vi "main_old.vi"() -> ()   [LabVIEW 2023]
uses:
  subVis/datas.ctl
  subVis/HologramInfo.ctl
  HoloPyLib/holoTracker.lvlib
  subVis/analyse_parameters.ctl
  <vilib>/Math Plots/3D Math Plots/3D Scatter/3D Scatter Datatype/3D Scatter Datatype.lvclass
  HoloPyLib/CCL_parameters.ctl
  HoloPyLib/parameters.ctl
  <vilib>/Math Plots/3D Math Plots/3D Scatter/3D Scatter Datatype/Public/Plot Helper (Vector).vi
  subVis/referencesBtns.ctl
  <vilib>/Math Plots/3D Math Plots/3D Scatter/3D Scatter XCtrl/3D Scatter.xctl
panel:
  out "Status":string
  in  "result tab":T1(tab)
  out "2D Picture":picture caption="Hologram"
  out "3D Scatter":refnum<class "3D Plot Datatype.lvclass">[](xcontrol)
  out "FEATURES":sgl[][](array[numeric])=[[0.0, 6.612585e-05, 1.9695788e-05, 1.0777613e-06, 1136.0], [0.0, 6.468655e-05, 2.2335455e-05, 1.0884105e-05, 10108.0], [0.0, 0.00015315457, 2.5819925e-05, 6.314848e-06, 8098.0], [0.0, 0.00014578222, 2.5758109e-05, 6.202794e-06, 6254.0], [0.0, 5.3788557e-05, 4.846046e-05, 1.6199401e-06, 4030.0], [0.0, 4.554296e-05, 5.2554697e-05, 2.3448233e-06, 5183.0], [0.0, 6.719615e-05, 0.00010475709, 9.479025e-06, 45705.0], [0.0, 0.0001519142, 0.000113882794, 3.5307496e-06, 7166.0], [0.0, 0.00014522657, 0.000117954936, 1.656648e-06, 2687.0], [0.0, 0.0001657626, 0.00017647912, 6.7820397e-06, 22008.0], [0.0, 0.0001543048, 0.00017526228, 4.2125926e-06, 4890.0], [0.0, 0.000108675, 0.00016782495, 4.2502693e-06, 6.0], [0.0, 5.2179905e-05, 4.8786325e-05, 1.0611426e-05, 896.0], [0.0, 7.633682e-05, 0.00010101719, 1.2997062e-05, 980.0], [0.0, 0.0001484, 0.000117425, 1.25e-05, 1.0], [0.0, 0.0001485656, 0.000115037496, 1.34489665e-05, 57.0], [0.0, 0.00014867843, 0.00011536141, 2.0105621e-05, 9059.0], [0.0, 4.993365e-05, 5.1556737e-05, 3.0146293e-05, 17286.0], [0.0, 0.00014947906, 2.572066e-05, 2.6544916e-05, 9378.0], [0.0, 3.406486e-05, 1.555056e-05, 3.0145982e-05, 9879.0], [0.0, 0.00014836973, 0.00013649464, 2.4943547e-05, 115.0], [0.0, 0.00010474305, 0.000167082, 3.4538934e-05, 11030.0], [0.0, 0.00016031138, 0.00017643355, 4.1315438e-05, 26224.0], [0.0, 4.673895e-05, 0.00013298314, 3.0840518e-05, 1181.0], [0.0, 4.4124776e-05, 0.000131255, 3.0545714e-05, 187.0], [0.0, 6.8812704e-05, 7.23215e-05, 3.4768887e-05, 4117.0], [0.0, 9.791127e-05, 5.2118266e-06, 3.6847057e-05, 2200.0], [0.0, 0.00017519953, 0.00015975515, 3.4322784e-05, 1209.0], [0.0, 0.00013256604, 3.5334786e-05, 3.941026e-05, 808.0], [0.0, 0.00013814989, 9.710776e-05, 3.901609e-05, 65.0], [0.0, 0.00016371529, 4.329701e-05, 4.3546614e-05, 2335.0]]
  in  "Tab Control":T2(tab)=enum."ACTIONS"
  in  "Holograms directory":path=path "C:/TRAVAIL/developpement/imagesHolo/1000im_manip3"
  in  "Test hologram path":path=path "C:/TRAVAIL/developpement/imagesHolo/1000im_manip3/100um_40x_int_.7ajmvz4e.000000.bmp"
  in  "Python version":string="3.10"
  in  "Analyse parameters":T3={"propagation"={"distance ini"=0.0, "number of planes"=200, "step"=5e-07, "Fourier BP filter (pix)"={"High pass (0=none)"=15.0, "Low Pass (0=none)"=125.0}}, "Focus"={"Type"=enum."SUM_OF_VARIANCE", "Sum size"=15}, "Remove mean Hologram"=FALSE, "CCL parameters"={"Threshold ( N x Standard deviation)"=10.0, "Connectivity"=enum."26", "min voxel"=1.0, "max voxel"=0.0}} {"CCL parameters"."max voxel" min=0.0 max=0.0; "CCL parameters"."min voxel" min=1.0 max=100.0; "CCL parameters"."Threshold ( N x Standard deviation)" min=1.0 max=100.0; "Focus"."Sum size" min=1 max=100; "propagation"."Fourier BP filter (pix)"."Low Pass (0=none)" format="%#_6f"; "propagation"."step" format="%#_6e"; "propagation"."distance ini" format="%#_6e"}
  in  "Holo parameters":T5={"wavelength"=6.6e-07, "optical index"=1.33, "Holo size X"=1024, "Holo size Y"=1024, "pixel size"=7e-06, "objective magnification"=40.0} {"wavelength" format="%#_6e"}
  in  "CANCEL_BATCH":bool
  in  "Batch parameters":T6
  in  "EXIT":bool
  in  "close HOLO":bool
  in  "findFeatures":bool
  in  "reconstruct&Focus":bool
  in  "removeMeanHolo":bool
  in  "openHOLO":bool
  in  "BATCH":bool
  out "dt(ms)":u32=190105
  in  "display\nsub-volume\n3 planes":bool
  in  "display_XY_SUM":bool
  in  "display_XZ_SUM":bool
  in  "display_YZ_SUM":bool
  in  "displayBinPlane":bool
  in  "TEST SUM BIN PLANE":bool
  in  "Plane number":u16=95
  in  "displayPlane":bool
  in  "displayXYMax":bool
  in  "displayXZMax":bool
  in  "displayYZMax":bool
  in  "displayHolo":bool
  in  "param":T7
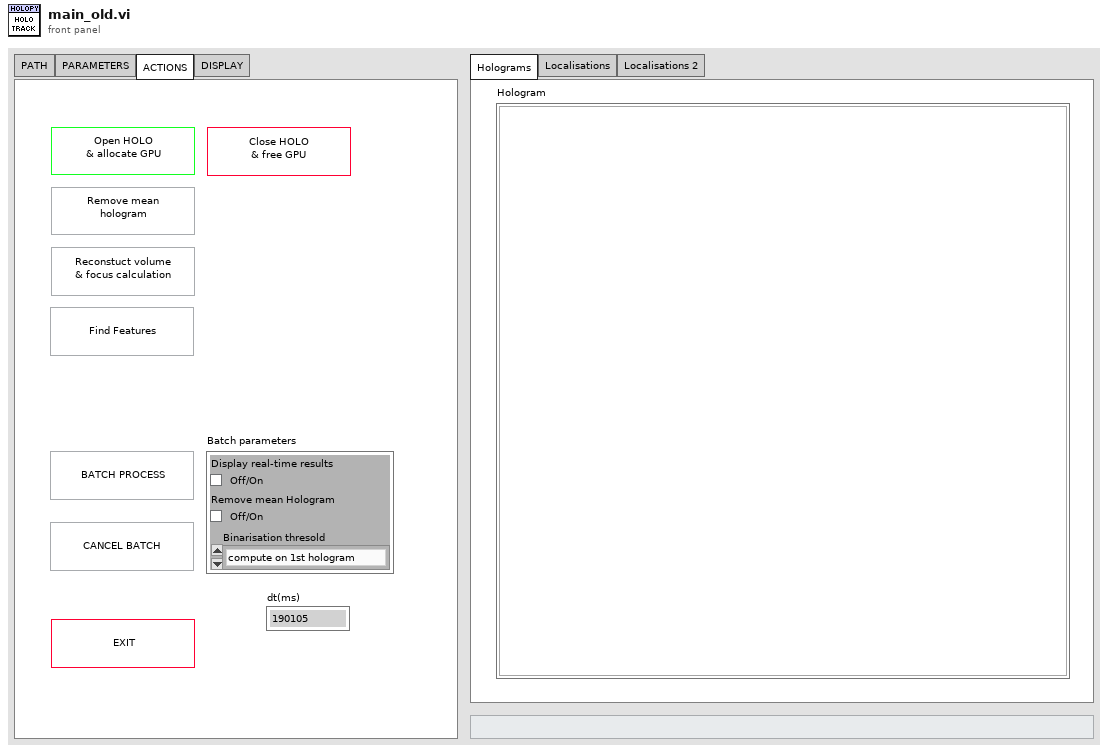
[diagram p1: front panel]
types:
  T1 = enum32{"Holograms", "Localisations", "Localisations 2"}
  T2 = enum32{"PATH", "PARAMETERS", "ACTIONS", "DISPLAY"}
  T3 = typedef "holoTracker.lvlib/analyse_parameters.ctl" = cluster{"propagation":cluster{"distance ini":dbl, "number of planes":i32, "step":dbl, "Fourier BP filter (pix)":cluster{"High pass (0=none)":dbl, "Low Pass (0=none)":dbl}}, "Focus":cluster{"Type":enum16{"SUM_OF_INTENSITY", "SUM_OF_LAPLACIAN", "SUM_OF_VARIANCE", "TENENGRAD"}, "Sum size":i32}, "Remove mean Hologram":bool, "CCL parameters":T4}
  T4 = typedef "CCL_parameters.ctl" = cluster{"Threshold ( N x Standard deviation)":dbl, "Connectivity":enum16{"6", "18", "26"}, "min voxel":dbl, "max voxel":dbl}
  T5 = typedef "holoTracker.lvlib/HologramInfo.ctl" = cluster{"wavelength":sgl, "optical index":sgl, "Holo size X":i32, "Holo size Y":i32, "pixel size":sgl, "objective magnification":sgl}
  T6 = cluster{"Display real-time results":bool, "Remove mean Hologram":bool, "Binarisation thresold ":enum16{"compute on 1st hologram", "compute on each hologram"}}
  T7 = cluster{"X":i32, "Y":i32, "Z":i32, "XYsize":i32, "ZSize":i32}
  T8 = typedef "referencesBtns.ctl" = cluster{"PythonVer":refnum<vi>, "Python/Environnement\npath":refnum<vi>, "HoloPath":refnum<vi>, "HoloDir":refnum<vi>, "Holo parameters":refnum<vi>, "Remove mean Hologram":refnum<vi>, "propagation":refnum<vi>, "Fourier BP filter (pix)":refnum<vi>, "Focus":refnum<vi>, "Batch thresold ":refnum<vi>, "CCL parameters":refnum<vi>, "testMode":refnum<vi>, "exitTestMode":refnum<vi>, "BATCH":refnum<vi>, "CANCEL_BATCH":refnum<vi>, "EXIT":refnum<vi>, "Plane number":refnum<vi>, "Display":refnum<vi>}
  T9 = typedef "datas.ctl" = cluster{"PythonSession":refnum<k35>, "Display":bool, "BinThreshold":sgl, "LIST HOLO BATCH":path[], "Display":sgl[][], "meanHolo":sgl[][], "FEATURES(µm)":sgl[][], "LabelPicture":string, "Status":string, "planeToDisplayFeatures":enum16{"XY", "XZ", "YZ"}, "State":enum16{"SESSION CLOSED", "WAIT", "TEST WAIT", "TEST IN PROGESS", "BATCH IN PROGRESS"}}
  T10 = typedef "parameters.ctl" = cluster{"Holo parameters":T5, "Analyse parameters":T3}
  T11 = cluster{"Test hologram path":path, "Display?":bool}
  T12 = cluster{"allocated?":bool, "reconstructed?":bool, "BATCH?":bool}
  T13 = cluster{"Holo":sgl[][], "XYFeatures(pix)":sgl[][], "FEATURES(µm)":sgl[][]}
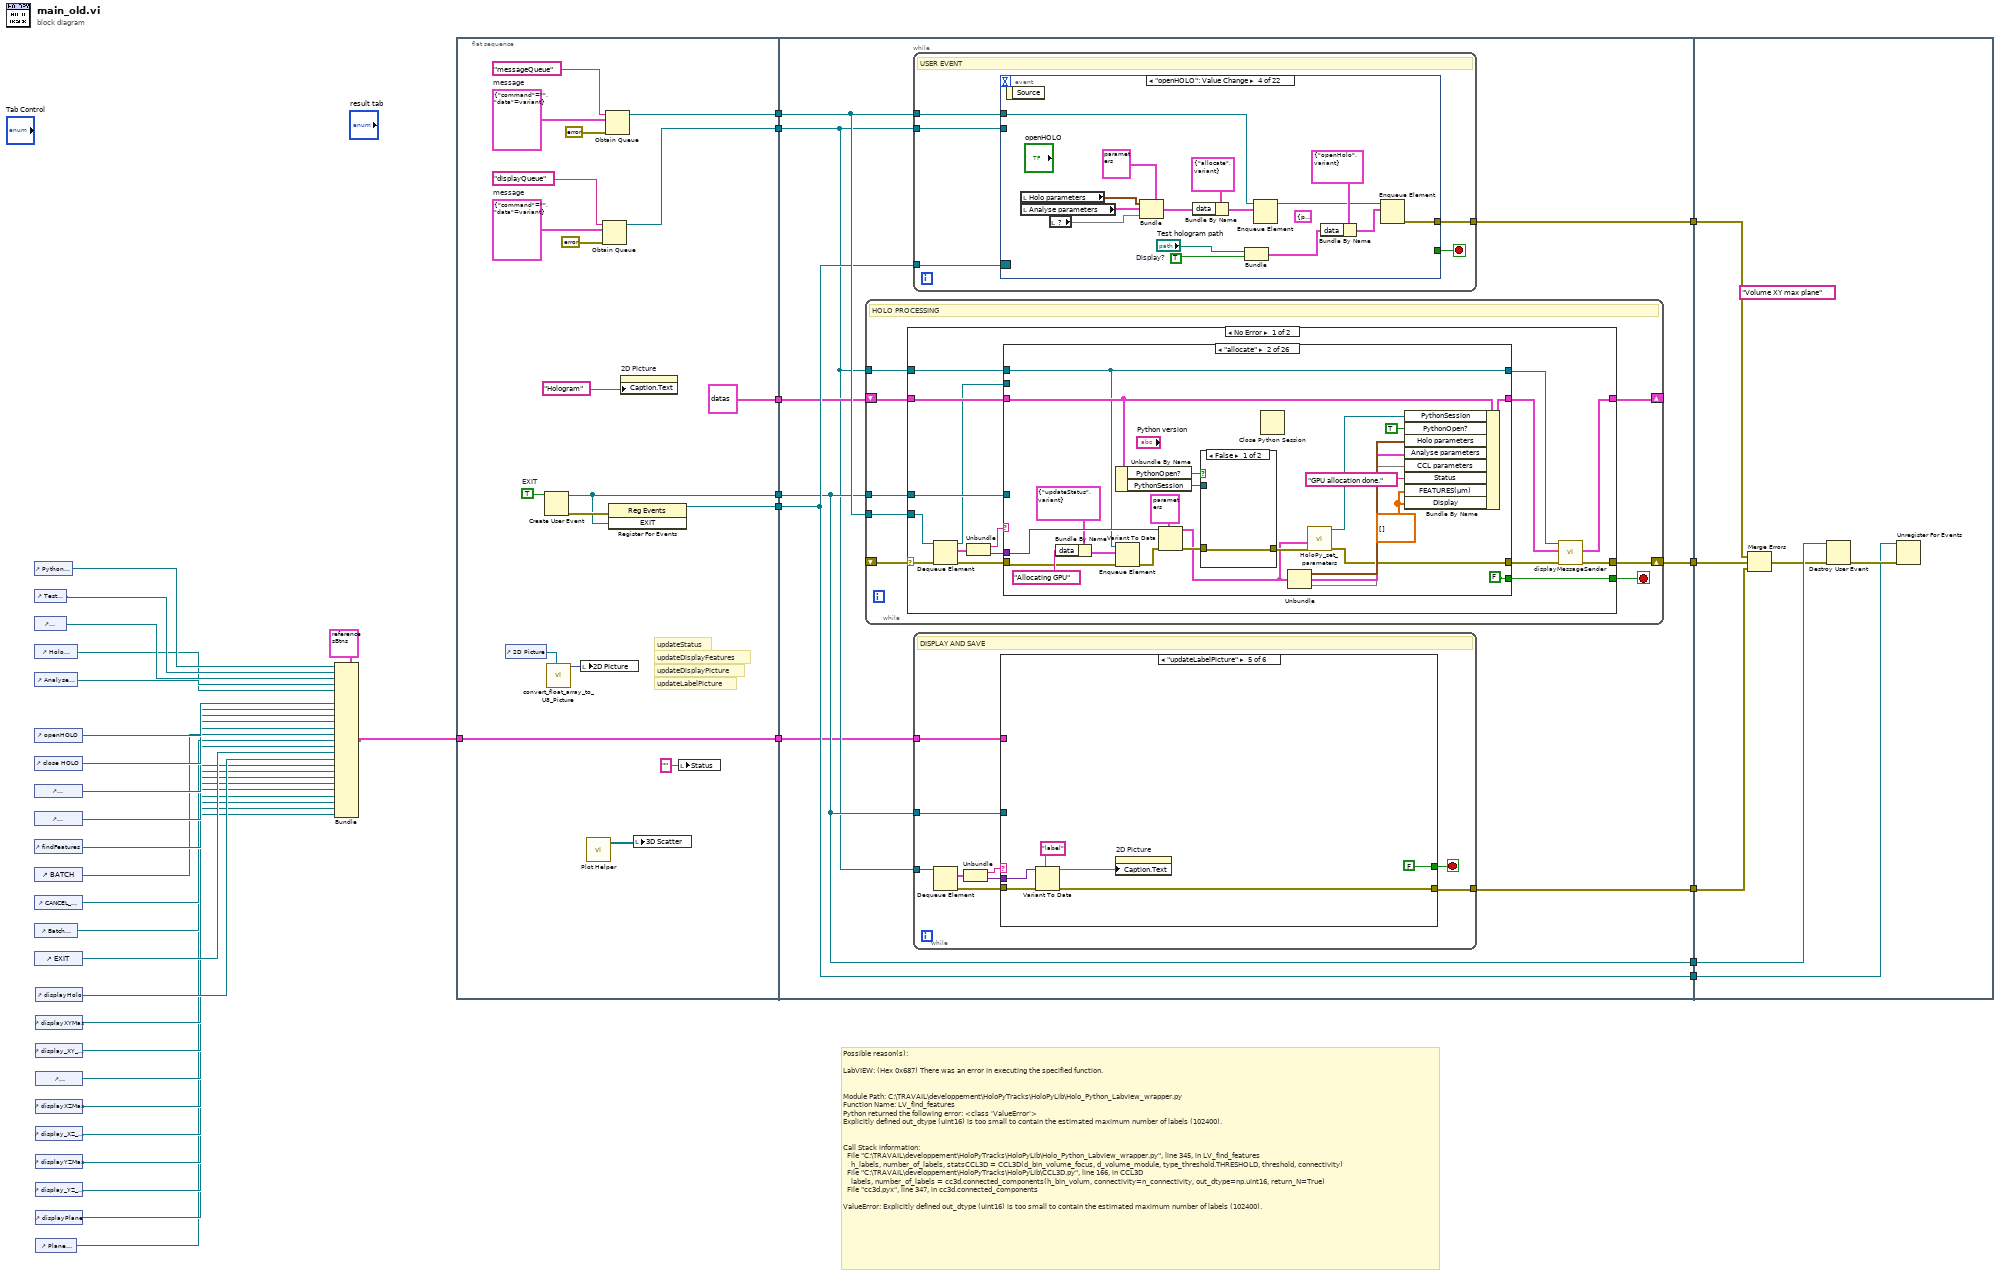
[diagram p0: block diagram]
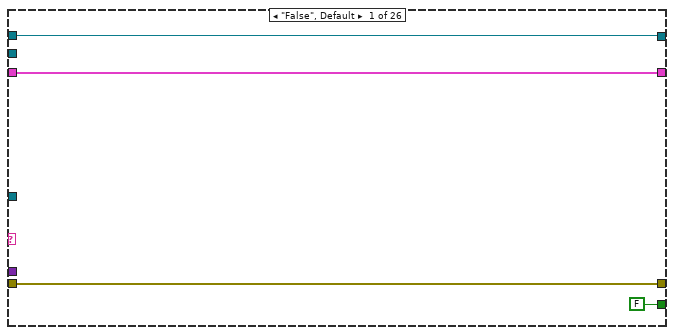
[diagram p2: hidden frame]
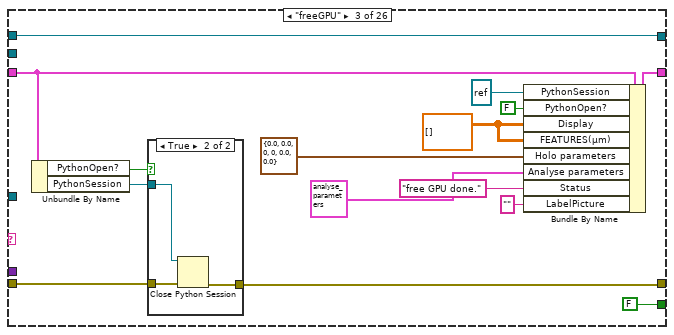
[diagram p4: hidden frame]
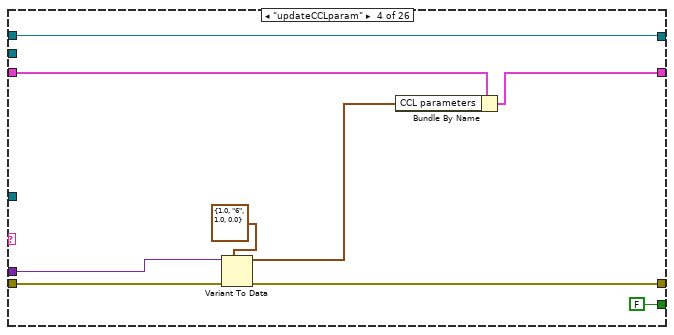
[diagram p6: hidden frame]
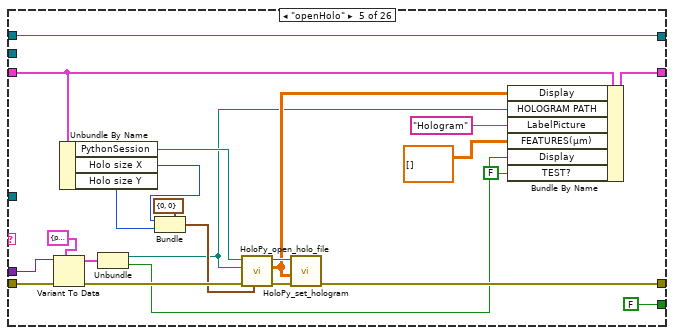
[diagram p7: hidden frame]
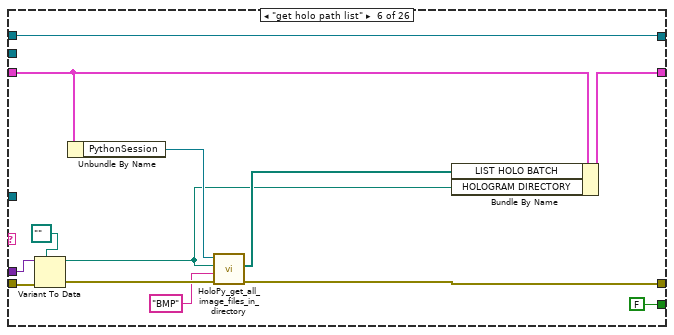
[diagram p8: hidden frame]
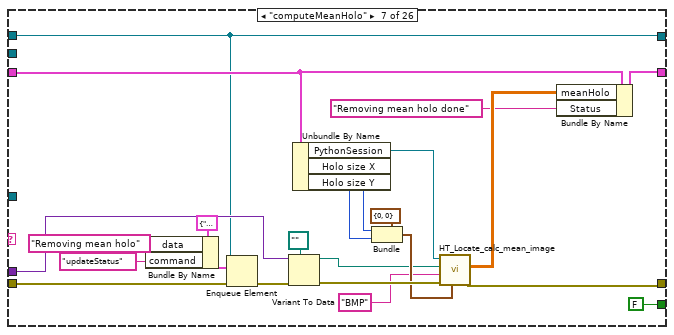
[diagram p9: hidden frame]
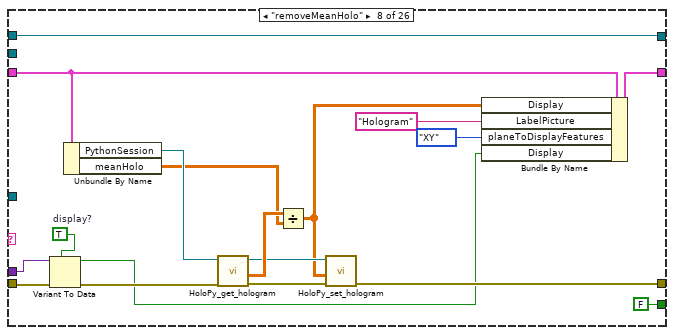
[diagram p10: hidden frame]
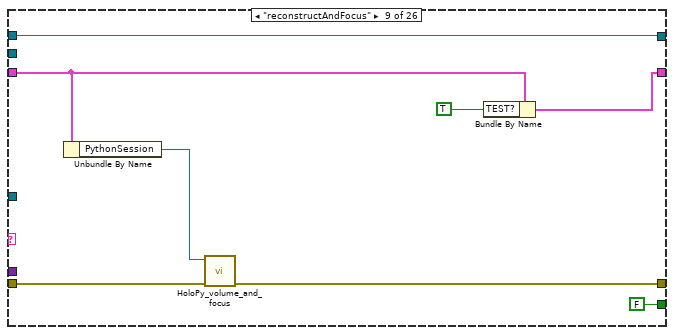
[diagram p11: hidden frame]
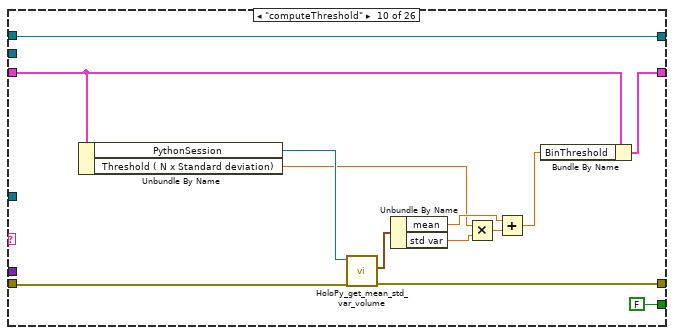
[diagram p12: hidden frame]
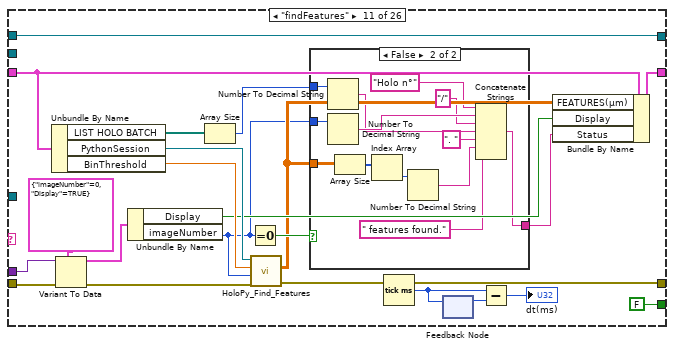
[diagram p13: hidden frame]
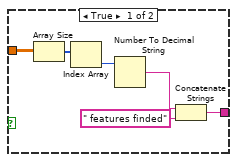
[diagram p14: hidden frame]
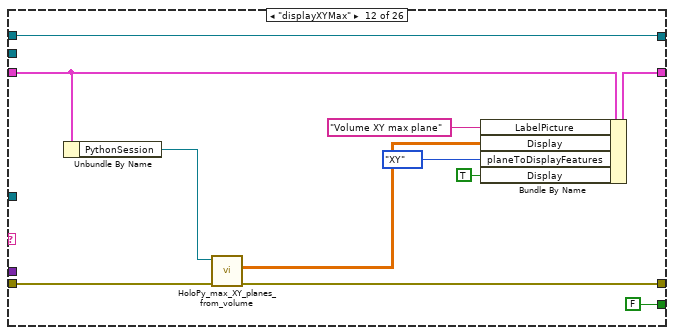
[diagram p15: hidden frame]
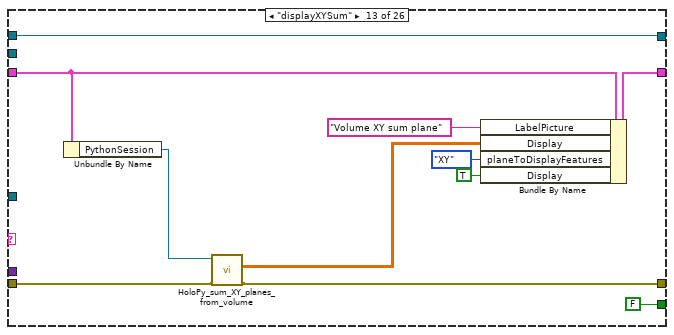
[diagram p16: hidden frame]
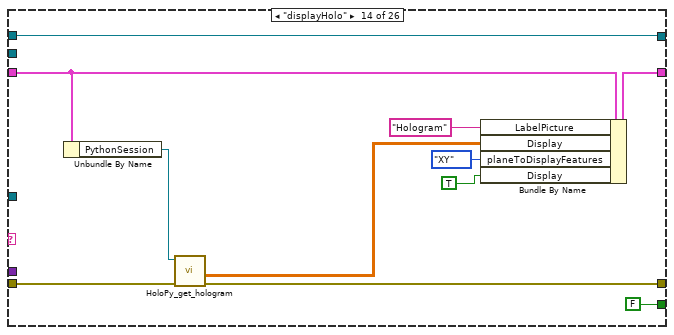
[diagram p17: hidden frame]
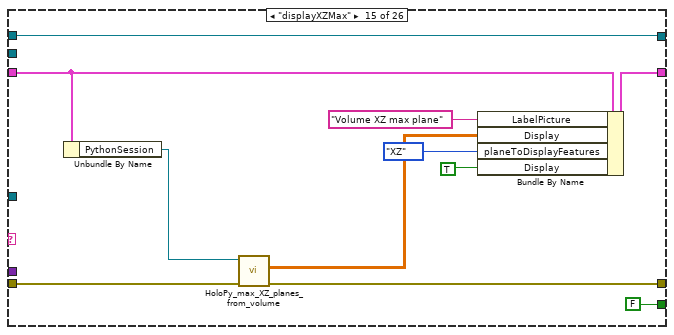
[diagram p18: hidden frame]
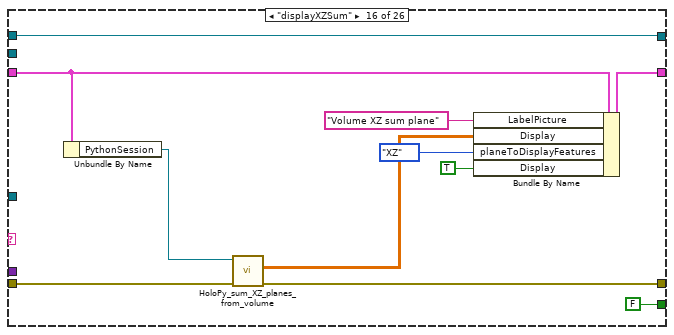
[diagram p19: hidden frame]
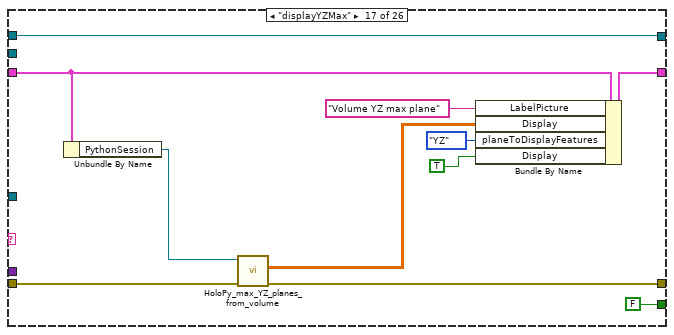
[diagram p20: hidden frame]
diagram:
  # "Possible reason(s):\n\nLabVIEW: (Hex 0x687) There was an error in executing the specified function.\n\n\nModule Path: C:\\TRAVAIL\\developpement\\HoloPyTracks\\HoloPyLib\\Holo_Python_Labview_wrapper.py\nFunction Name: LV_find_features\nPython returned the following error: <class 'ValueError'>\nExplicitly defined out_dtype (uint16) is too small to contain the estimated maximum number of labels (102400).\n\n\nCall Stack information:\n  File \"C:\\TRAVAIL\\developpement\\HoloPyTracks\\HoloPyLib\\Holo_Python_Labview_wrapper.py\", line 345, in LV_find_features\n    h_labels, number_of_labels, statsCCL3D = CCL3D(d_bin_volume_focus, d_volume_module, type_threshold.THRESHOLD, threshold, connectivity)\n  File \"C:\\TRAVAIL\\developpement\\HoloPyTracks\\HoloPyLib\\CCL3D.py\", line 166, in CCL3D\n    labels, number_of_labels = cc3d.connected_components(h_bin_volum, connectivity=n_connectivity, out_dtype=np.uint16, return_N=True)\n  File \"cc3d.pyx\", line 347, in cc3d.connected_components\n\nValueError: Explicitly defined out_dtype (uint16) is too small to contain the estimated maximum number of labels (102400)."
  n1 = control-ref of="Python version"() -> (w28:refnum<vi>)
  n2 = control-ref of="Test hologram path"() -> (w27:refnum<vi>)
  n3 = control-ref of="Holograms directory"() -> (w26:refnum<vi>)
  n4 = control-ref of="Holo parameters"() -> (w25:refnum<vi>)
  n5 = control-ref of="Analyse parameters"() -> (w24:refnum<vi>)
  n6 = control-ref of="openHOLO"() -> (w22:refnum<vi>)
  n7 = control-ref of="close HOLO"() -> (w21:refnum<vi>)
  n8 = control-ref of="removeMeanHolo"() -> (w20:refnum<vi>)
  n9 = control-ref of="reconstruct&Focus"() -> (w19:refnum<vi>)
  n10 = control-ref of="findFeatures"() -> (w18:refnum<vi>)
  n11 = control-ref of="BATCH"() -> (w17:refnum<vi>)
  n12 = control-ref of="CANCEL_BATCH"() -> (w16:refnum<vi>)
  n13 = control-ref of="Batch parameters"() -> (w15:refnum<vi>)
  n14 = control-ref of="EXIT"() -> (w14:refnum<vi>)
  n15 = control-ref of="displayHolo"() -> (w13:refnum<vi>)
  n16 = control-ref of="displayXYMax"() -> (w12:refnum<vi>)
  n17 = control-ref of="display_XY_SUM"() -> (w11:refnum<vi>)
  n18 = control-ref of="displayBinPlane"() -> (w10:refnum<vi>)
  n19 = control-ref of="displayXZMax"() -> (w9:refnum<vi>)
  n20 = control-ref of="display_XZ_SUM"() -> (w8:refnum<vi>)
  n21 = control-ref of="displayYZMax"() -> (w7:refnum<vi>)
  n22 = control-ref of="display_YZ_SUM"() -> (w6:refnum<vi>)
  n23 = control-ref of="displayPlane"() -> (w5:refnum<vi>)
  n24 = control-ref of="Plane number"() -> (w4:refnum<vi>)
  n25 = Bundle(cluster=T8 {"PythonVer"=refnum, "Python/Environnement\npath"=refnum, "HoloPath"=refnum, "HoloDir"=refnum, "Holo parameters"=refnum, "Remove mean Hologram"=refnum, "propagation"=refnum, "Fourier BP filter (pix)"=refnum, "Focus"=refnum, "Batch thresold "=refnum, "CCL parameters"=refnum, "testMode"=refnum, "exitTestMode"=refnum, "BATCH"=refnum, "CANCEL_BATCH"=refnum, "EXIT"=refnum, "Plane number"=refnum, "Display"=refnum} ("output cluster"), w28, w27, w26, w25, w24, w22, w21, w20, w19, w18, w17, w16, w15, w14, w13, w12, w11, w10, w9, w8, w7, w6, w5, w4) -> (w1:T8, w23:refnum<vi>)
  n26 = flat-sequence {
    tunnel: [w55] -> w38
    tunnel: [w51] -> w37
    tunnel: [w50] -> w36
    tunnel: [w46] -> w35
    tunnel: [T9 {"PythonSession"=refnum, "Display"=FALSE, "BinThreshold"=0.0, "LIST HOLO BATCH"=[], "Display"=[], "meanHolo"=[], "FEATURES(µm)"=[], "LabelPicture"="", "Status"="", "planeToDisplayFeatures"=enum."XY", "State"=enum."WAIT"}] -> w34
    tunnel: [w39] -> w2
    tunnel: w1 -> [w39]
    tunnel: w38 -> [w66]
    tunnel: w37 -> [w63]
    tunnel: w36 -> [w65]
    tunnel: w35 -> [w61]
    tunnel: w34 -> [w62]
    tunnel: [w65] -> w33
    tunnel: [w63] -> w32
    tunnel: [w64] -> w31
    tunnel: [w60] -> w30
    tunnel: [w59] -> w29
    tunnel: w2 -> [w58]
    tunnel: w33 -> [w695]
    tunnel: w32 -> [w694]
    tunnel: w31 -> [w691]
    tunnel: w30 -> [w693]
    tunnel: w29 -> [w692]
    frame #0 {
      w48 = cluster{"command":string, "data":variant} {"command"="", "data"=variant}  # message
      w53 = TRUE  # EXIT
      w56 = cluster{"command":string, "data":variant} {"command"="", "data"=variant}  # message
      # "updateDisplayFeatures"
      # "updateLabelPicture"
      # "updateDisplayPicture"
      # "updateStatus"
      n27 = control-ref of="2D Picture"() -> (w44:refnum<vi>)
      n28 = Create User Event(user event datatype=w53) -> (user event=w51:refnum<user-event>, error out=w52:errorcluster)  [unwired: 1 in]
      n29 = call "convert_float_array_to_U8_Picture.vi"("Pict Refnum"=w44) -> ("new picture"=w43:picture)  [unwired: 9 in, 1 out]
      n30 = local write "2D Picture"(w43) -> ()
      n31 = call-poly <vilib>:"Plot Helper.vi"() -> ("3D Plot lvclass Array out"=w40:refnum<class "3D Plot Datatype.lvclass">[])  [unwired: 6 in, 5 out]
      n32 = Obtain Queue(name (unnamed)="displayQueue", element data type=w48, error in (no error)=errorcluster {"status"=FALSE, "code"=0, "source"=""}) -> (queue out=w46:refnum<queue>)  [unwired: 2 in, 2 out]
      n33 = Obtain Queue(name (unnamed)="messageQueue", element data type=w56, error in (no error)=errorcluster {"status"=FALSE, "code"=0, "source"=""}) -> (queue out=w55:refnum<queue>)  [unwired: 2 in, 2 out]
      n34 = register-events(error in=w52, w51) -> (reference out=w50:refnum<event-registration>)  [unwired: 1 in, 1 out]
      n35 = property on="2D Picture" class="Pict"("Caption.Text"="Hologram" ("Label.Text")) -> ()  [unwired: 2 in, 2 out]
      n36 = local write "3D Scatter"(w40) -> ()
      n37 = local write "Status"("" ("Status")) -> ()
    }
    frame #1 {
      n38 = while {
        tunnel: w66 -> [w74]
        tunnel: w63 -> [w72]
        shift-right: [w70] -> _
        shift-left: w62 -> [w71]
        tunnel: w61 -> [w69]
        shift-right: [w68] -> w59
        shift-left: _ -> [w67]
        stop <- w73 stop-if-true
        # "HOLO PROCESSING"
        n39 = case shown="No Error" w67 {
          selector: w67 -> [w80 w489]
          tunnel: w74 -> [w90 w490]
          tunnel: [w85 FALSE] -> w73
          tunnel: w72 -> [w84 _]
          tunnel: w71 -> [w83 w485]
          tunnel: [w75 w485] -> w70
          tunnel: w69 -> [w82 _]
          tunnel: [w77 errorcluster {"status"=FALSE, "code"=0, "source"=""} ("error out")] -> w68
          frame No Error {
            n40 = Dequeue Element(queue=w90, error in (no error)=w80) -> (queue out=w81:refnum<queue>, element=w88:cluster{"command":string, "data":variant}, error out=w89:errorcluster)  [unwired: 1 in, 1 out]
            n41 = Unbundle(w88) -> ("command"=w87:string, "data"=w86:variant)
            n42 = case shown="\"allocate\"" w87 {
              tunnel: w89 -> [w92 w98 w128 w146 w169 w182 w190 w211 w231 w239 w266 w296 w302 w313 w324 w335 w346 w357 w369 w394 w411 w415 w433 w443 w467 w476]
              tunnel: w86 -> [_ w117 _ w145 w168 w181 w205 w210 _ _ w265 _ _ _ _ _ _ _ w368 w393 w410 _ w432 _ w466 _]
              tunnel: [FALSE FALSE FALSE FALSE FALSE FALSE FALSE FALSE FALSE FALSE FALSE FALSE FALSE FALSE FALSE FALSE FALSE FALSE FALSE FALSE FALSE FALSE FALSE FALSE FALSE TRUE] -> w85
              tunnel: w84 -> [_ _ _ _ _ _ _ _ _ _ _ _ _ _ _ _ _ _ _ _ _ _ _ _ _ w479]
              tunnel: w83 -> [w93 w115 w132 w142 w161 w179 w197 w218 w227 w237 w257 w292 w306 w317 w328 w339 w350 w361 w376 w389 w409 w422 w425 w451 w460 w471]
              tunnel: [w93 w116 w133 w141 w160 w180 w196 w216 w226 w236 w255 w291 w305 w316 w327 w338 w349 w360 w375 w388 w408 w421 w424 w452 w460 w470] -> w79
              tunnel: w82 -> [w91 w96 w122 w139 w153 w171 w184 w215 w229 w233 w258 w294 w307 w318 w329 w340 w351 w362 w377 w387 w407 w420 w427 w441 w458 w472]
              tunnel: [w92 w103 w124 w143 w151 w174 w186 w214 w228 w238 w256 w293 w299 w312 w321 w334 w345 w356 w372 w381 w398 w419 w429 w438 w463 w473] -> w76
              tunnel: w81 -> [_ _ _ _ _ _ _ _ _ _ _ _ _ _ _ _ _ _ _ _ _ _ w434 w444 _ _]
              tunnel: [w91 w96 w122 w139 w153 w171 w184 w215 w229 w233 w258 w294 w307 w318 w329 w340 w351 w362 w377 w387 w407 w420 w427 w441 w458 w472] -> w78
              frame "False", Default {
              }
              frame "allocate" {
                w101 = sgl[][] [] ("FEATURES(µm)")
                n43 = Bundle By Name(cluster=cluster{"command":string, "data":variant} {"command"="updateStatus", "data"=variant} ("element"), "data"="Allocating GPU" ("command")) -> (w95:cluster{"command":string, "data":variant})
                n44 = Unbundle By Name(w115) -> ("PythonOpen?"=w113:bool, "PythonSession"=w112:refnum<k35>)
                n45 = Enqueue Element(queue=w96, element=w95, error in (no error)=w98) -> (error out=w97:errorcluster)  [unwired: 1 in, 2 out]
                n46 = Variant To Data(error in=w97, type=T10 {"Holo parameters"={"wavelength"=0.0, "optical index"=0.0, "Holo size X"=0, "Holo size Y"=0, "pixel size"=0.0, "objective magnification"=0.0}, "Analyse parameters"={"propagation"={"distance ini"=0.0, "number of planes"=0, "step"=0.0, "Fourier BP filter (pix)"={"High pass (0=none)"=0.0, "Low Pass (0=none)"=0.0}}, "Focus"={"Type"=enum."SUM_OF_INTENSITY", "Sum size"=0}, "Remove mean Hologram"=FALSE, "CCL parameters"={"Threshold ( N x Standard deviation)"=10.0, "Connectivity"=enum."26", "min voxel"=1.0, "max voxel"=0.0}}} ("Parameters"), Variant=w117) -> (data=w105:T10, error out=w114:errorcluster)
                n47 = case shown="False" w113 {
                  tunnel: w114 -> [w119 _]
                  tunnel: w112 -> [_ _]
                  tunnel: [w119 _] -> w111
                  frame False {
                  }
                  frame True {
                  }
                }
                n48 = Close Python Session() -> ()  [unwired: 2 in, 1 out]
                n49 = Unbundle(w105) -> (w108:T5, w107:T3, w104)
                n50 = call "HoloPy_set_parameters.vi"("error in (no error)"=w111, 9:w105) -> ("error out"=w103:errorcluster, "Refnum out"=w110:refnum<k35>)  [unwired: 7 in, 1 out]
                n51 = Bundle By Name(cluster=w115, "PythonSession"=w110, "PythonOpen?"=TRUE ("allocated?"), "Holo parameters"=w108, "Analyse parameters"=w107, "CCL parameters"=w104, "Status"="GPU allocation done." ("command"), "FEATURES(µm)"=w101, "Display"=w101) -> (w116:T9)
              }
              frame "freeGPU" {
                w120 = sgl[][] [] ("Holo")
                n52 = Unbundle By Name(w132) -> ("PythonOpen?"=w131:bool, "PythonSession"=w130:refnum<k35>)
                n53 = case shown="True" w131 {
                  tunnel: w128 -> [w135 w138]
                  tunnel: w130 -> [_ w137]
                  tunnel: [w135 w136] -> w124
                  frame False {
                  }
                  frame True {
                    n54 = Close Python Session(session in=w137, error in=w138) -> (11:w136:errorcluster)
                  }
                }
                n55 = Bundle By Name(cluster=w132, "PythonSession"=refnum<k35> refnum, "PythonOpen?"=FALSE ("allocated?"), "Display"=w120, "FEATURES(µm)"=w120, "Holo parameters"=T5 {"wavelength"=0.0, "optical index"=0.0, "Holo size X"=0, "Holo size Y"=0, "pixel size"=0.0, "objective magnification"=0.0}, "Analyse parameters"=T3 {"propagation"={"distance ini"=0.0, "number of planes"=0, "step"=0.0, "Fourier BP filter (pix)"={"High pass (0=none)"=0.0, "Low Pass (0=none)"=0.0}}, "Focus"={"Type"=enum."SUM_OF_INTENSITY", "Sum size"=1}, "Remove mean Hologram"=FALSE, "CCL parameters"={"Threshold ( N x Standard deviation)"=10.0, "Connectivity"=enum."26", "min voxel"=1.0, "max voxel"=0.0}}, "Status"="free GPU done." ("command"), "LabelPicture"="" ("command")) -> (w133:T9)
              }
              frame "updateCCLparam" {
                n56 = Variant To Data(error in=w146, type=T4 {"Threshold ( N x Standard deviation)"=1.0, "Connectivity"=enum."6", "min voxel"=1.0, "max voxel"=0.0} ("CCL parameters"), Variant=w145) -> (data=w140:T4, error out=w143:errorcluster)
                n57 = Bundle By Name(cluster=w142, "CCL parameters"=w140) -> (w141:T9)
              }
              frame "openHolo" {
                n58 = Variant To Data(error in=w169, type=T11 {"Test hologram path"=path "", "Display?"=FALSE} ("openHolo"), Variant=w168) -> (data=w155:T11, error out=w166:errorcluster)
                n59 = Unbundle By Name(w161) -> ("PythonSession"=w167:refnum<k35>, "Holo size X"=w163:i32, "Holo size Y"=w162:i32)
                n60 = Unbundle(w155) -> ("Test hologram path"=w154:path, "Display?"=w149:bool)
                n61 = Bundle(cluster=cluster{"image_size_X":i32, "image_size_Y":i32} {"image_size_X"=0, "image_size_Y"=0} ("imageSize"), "image_size_X"=w163, "image_size_Y"=w162) -> (w164:cluster{"image_size_X":i32, "image_size_Y":i32})
                n62 = call "HoloPy_open_holo_file.vi"("imageSize"=w164, "error in (no error)"=w166, "image path"=w154, "Refnum in"=w167) -> ("error out"=w159:errorcluster, "Array"=w157:sgl[][], "Refnum out"=w158:refnum<k35>)  [unwired: 5 in]
                n63 = call "HoloPy_set_hologram.vi"("error in (no error)"=w159, "HOLO_array"=w157, "Refnum in"=w158) -> ("error out"=w151:errorcluster)  [unwired: 6 in, 2 out]
                n64 = Bundle By Name(cluster=w161, "Display"=w157, "HOLOGRAM PATH"=w154, "LabelPicture"="Hologram" ("Label.Text"), "FEATURES(µm)"=sgl[][] [], "Display"=w149, "TEST?"=FALSE ("reconstructed?")) -> (w160:T9)
              }
              frame "get holo path list" {
                n65 = Variant To Data(error in=w182, type=path "" ("Holograms directory"), Variant=w181) -> (data=w173:path, error out=w178:errorcluster)
                n66 = Unbundle By Name(w179) -> ("PythonSession"=w177:refnum<k35>)
                n67 = call "HoloPy_get_all_image_files_in_directory.vi"("error in (no error)"=w178, "file_extension"="BMP", "holo directory"=w173, "Refnum in"=w177) -> ("error out"=w174:errorcluster, "path"=w175:path[])  [unwired: 5 in, 1 out]
                n68 = Bundle By Name(cluster=w179, "LIST HOLO BATCH"=w175, "HOLOGRAM DIRECTORY"=w173) -> (w180:T9)
              }
              frame "computeMeanHolo" {
                n69 = Bundle By Name(cluster=cluster{"command":string, "data":variant} {"command"="", "data"=variant} ("element"), "data"="Removing mean holo" ("command"), "command"="updateStatus") -> (w192:cluster{"command":string, "data":variant})
                n70 = Enqueue Element(queue=w184, element=w192, error in (no error)=w190) -> (error out=w189:errorcluster)  [unwired: 1 in, 2 out]
                n71 = Variant To Data(error in=w189, type=path "" ("Holograms directory"), Variant=w205) -> (data=w187:path, error out=w201:errorcluster)
                n72 = Unbundle By Name(w197) -> ("PythonSession"=w199:refnum<k35>, "Holo size X"=w203:i32, "Holo size Y"=w202:i32)
                n73 = Bundle(cluster=cluster{"image_size_X":i32, "image_size_Y":i32} {"image_size_X"=0, "image_size_Y"=0} ("imageSize"), "image_size_X"=w203, "image_size_Y"=w202) -> (w200:cluster{"image_size_X":i32, "image_size_Y":i32})
                n74 = call "HT_Locate_calc_mean_image.vi"("imageSize"=w200, "error in (no error)"=w201, "imageFileExtension"="BMP", "directory path"=w187, "Refnum in"=w199) -> ("error out"=w186:errorcluster, "Array"=w195:sgl[][])  [unwired: 4 in, 1 out]
                n75 = Bundle By Name(cluster=w197, "meanHolo"=w195, "Status"="Removing mean holo done" ("command")) -> (w196:T9)
              }
              frame "removeMeanHolo" {
                w209 = TRUE  # display?
                n76 = Variant To Data(error in=w211, type=w209, Variant=w210) -> (data=w207:bool, error out=w208:errorcluster)
                n77 = Unbundle By Name(w218) -> ("PythonSession"=w220:refnum<k35>, "meanHolo"=w219:sgl[][])
                n78 = call "HoloPy_get_hologram.vi"("error in (no error)"=w208, "Refnum in"=w220) -> ("error out"=w222:errorcluster, "HOLO_array"=w223:sgl[][], "Refnum out"=w221:refnum<k35>)  [unwired: 7 in]
                n79 = Divide(x=w223, y=w219) -> (x/y=w217:sgl[][])
                n80 = call "HoloPy_set_hologram.vi"("error in (no error)"=w222, "HOLO_array"=w217, "Refnum in"=w221) -> ("error out"=w214:errorcluster)  [unwired: 6 in, 2 out]
                n81 = Bundle By Name(cluster=w218, "Display"=w217, "LabelPicture"="Hologram", "planeToDisplayFeatures"=enum16{"XY", "XZ", "YZ"}."XY", "Display"=w207) -> (w216:T9)
              }
              frame "reconstructAndFocus" {
                n82 = Unbundle By Name(w227) -> ("PythonSession"=w230:refnum<k35>)
                n83 = call "HoloPy_volume_and_focus.vi"("error in (no error)"=w231, "Refnum in"=w230) -> ("error out"=w228:errorcluster)  [unwired: 7 in, 2 out]
                n84 = Bundle By Name(cluster=w227, "TEST?"=TRUE ("reconstructed?")) -> (w226:T9)
              }
              frame "computeThreshold" {
                n85 = Unbundle By Name(w237) -> ("PythonSession"=w244:refnum<k35>, "Threshold ( N x Standard deviation)"=w234:dbl)
                n86 = call "HoloPy_get_mean_std_var_volume.vi"("error in (no error)"=w239, "Refnum in"=w244) -> ("error out"=w238:errorcluster, "data volume"=w243:cluster{"mean":dbl, "std var":dbl})  [unwired: 7 in, 1 out]
                n87 = Unbundle By Name(w243) -> ("mean"=w240:dbl, "std var"=w242:dbl)
                n88 = Multiply(x=w234, y=w242) -> (x*y=w241:dbl)
                n89 = Add(x=w240, y=w241) -> (x+y=w235:dbl)
                n90 = Bundle By Name(cluster=w237, "BinThreshold"=w235) -> (w236:T9)
              }
              frame "findFeatures" {
                n91 = Unbundle By Name(w257) -> ("LIST HOLO BATCH"=w251:path[], "PythonSession"=w263:refnum<k35>, "BinThreshold"=w264:sgl)
                n92 = Variant To Data(error in=w266, type=cluster{"imageNumber":u32, "Display":bool} {"imageNumber"=0, "Display"=TRUE}, Variant=w265) -> (data=w253:cluster{"imageNumber":u32, "Display":bool}, error out=w262:errorcluster)
                n93 = Unbundle By Name(w253) -> ("Display"=w252:bool, "imageNumber"=w247:u32)
                n94 = Array Size(array=w251) -> (size(s)=w246:i32)
                n95 = Equal To 0?(x=w247) -> (x = 0?=w250:bool)
                n96 = call "HoloPy_Find_Features.vi"("error in (no error)"=w262, "imageNumber"=w247, "Threshold"=w264, "Refnum in"=w263) -> ("error out"=w256:errorcluster, "FEATURES(µm)"=w249:sgl[][])  [unwired: 5 in, 1 out]
                n97 = case shown="False" w250 {
                  tunnel: w249 -> [w273 w286]
                  tunnel: [w268 w274] -> w248
                  tunnel: w247 -> [_ w282]
                  tunnel: w246 -> [_ w283]
                  frame True {
                    n98 = Array Size(array=w273) -> (size(s)=w272:i32[])
                    n99 = Index Array(array=w272) -> (element=w271:i32)  [unwired: 1 in]
                    n100 = Number To Decimal String(number=w271) -> (decimal integer string=w269:string)  [unwired: 1 in]
                    n101 = Concatenate Strings(w269, " features finded") -> (w268:string)
                  }
                  frame False {
                    n102 = Number To Decimal String(number=w283) -> (decimal integer string=w278:string)  [unwired: 1 in]
                    n103 = Number To Decimal String(number=w282) -> (decimal integer string=w280:string)  [unwired: 1 in]
                    n104 = Array Size(array=w286) -> (size(s)=w285:i32[])
                    n105 = Index Array(array=w285) -> (element=w284:i32)  [unwired: 1 in]
                    n106 = Number To Decimal String(number=w284) -> (decimal integer string=w276:string)  [unwired: 1 in]
                    n107 = Concatenate Strings("Holo n°", w280, "/", w278, ". " ("string"), w276, " features found.") -> (w274:string)
                  }
                }
                n108 = Tick Count (ms)() -> (millisecond timer value=w260:u32)
                n109 = feedback-in #1(w260) -> ()
                n110 = feedback #1() -> (w261:u32)  [unwired: 1 in]
                n111 = Subtract(x=w260, y=w261) -> (x-y=→"dt(ms)":u32)
                n112 = Bundle By Name(cluster=w257, "FEATURES(µm)"=w249, "Display"=w252, "Status"=w248) -> (w255:T9)
              }
              frame "displayXYMax" {
                n113 = Unbundle By Name(w292) -> ("PythonSession"=w295:refnum<k35>)
                n114 = call "HoloPy_max_XY_planes_from_volume.vi"("error in (no error)"=w296, "Refnum in"=w295) -> ("error out"=w293:errorcluster, "XY Plane"=w289:sgl[][])  [unwired: 7 in, 1 out]
                n115 = Bundle By Name(cluster=w292, "LabelPicture"="Volume XY max plane" ("Label.Text"), "Display"=w289, "planeToDisplayFeatures"=enum16{"XY", "XZ", "YZ"}."XY", "Display"=TRUE) -> (w291:T9)
              }
              frame "displayXYSum" {
                n116 = Unbundle By Name(w306) -> ("PythonSession"=w301:refnum<k35>)
                n117 = call "HoloPy_sum_XY_planes_from_volume.vi"("error in (no error)"=w302, "Refnum in"=w301) -> ("error out"=w299:errorcluster, "XY Plane"=w300:sgl[][])  [unwired: 7 in, 1 out]
                n118 = Bundle By Name(cluster=w306, "LabelPicture"="Volume XY sum plane" ("Label.Text"), "Display"=w300, "planeToDisplayFeatures"=enum16{"XY", "XZ", "YZ"}."XY", "Display"=TRUE) -> (w305:T9)
              }
              frame "displayHolo" {
                n119 = Unbundle By Name(w317) -> ("PythonSession"=w311:refnum<k35>)
                n120 = call "HoloPy_get_hologram.vi"("error in (no error)"=w313, "Refnum in"=w311) -> ("error out"=w312:errorcluster, "HOLO_array"=w310:sgl[][])  [unwired: 7 in, 1 out]
                n121 = Bundle By Name(cluster=w317, "LabelPicture"="Hologram" ("Label.Text"), "Display"=w310, "planeToDisplayFeatures"=enum16{"XY", "XZ", "YZ"}."XY", "Display"=TRUE) -> (w316:T9)
              }
              frame "displayXZMax" {
                n122 = Unbundle By Name(w328) -> ("PythonSession"=w323:refnum<k35>)
                n123 = call "HoloPy_max_XZ_planes_from_volume.vi"("error in (no error)"=w324, "Refnum in"=w323) -> ("error out"=w321:errorcluster, "XZ Plane"=w322:sgl[][])  [unwired: 7 in, 1 out]
                n124 = Bundle By Name(cluster=w328, "LabelPicture"="Volume XZ max plane" ("Label.Text"), "Display"=w322, "planeToDisplayFeatures"=enum16{"XY", "XZ", "YZ"}."XZ", "Display"=TRUE) -> (w327:T9)
              }
              frame "displayXZSum" {
                n125 = Unbundle By Name(w339) -> ("PythonSession"=w332:refnum<k35>)
                n126 = call "HoloPy_sum_XZ_planes_from_volume.vi"("error in (no error)"=w335, "Refnum in"=w332) -> ("error out"=w334:errorcluster, "XZ Plane"=w333:sgl[][])  [unwired: 7 in, 1 out]
                n127 = Bundle By Name(cluster=w339, "LabelPicture"="Volume XZ sum plane" ("Label.Text"), "Display"=w333, "planeToDisplayFeatures"=enum16{"XY", "XZ", "YZ"}."XZ", "Display"=TRUE) -> (w338:T9)
              }
              frame "displayYZMax" {
                n128 = Unbundle By Name(w350) -> ("PythonSession"=w343:refnum<k35>)
                n129 = call "HoloPy_max_YZ_planes_from_volume.vi"("error in (no error)"=w346, "Refnum in"=w343) -> ("error out"=w345:errorcluster, "YZ Plane"=w344:sgl[][])  [unwired: 7 in, 1 out]
                n130 = Bundle By Name(cluster=w350, "LabelPicture"="Volume YZ max plane" ("Label.Text"), "Display"=w344, "planeToDisplayFeatures"=enum16{"XY", "XZ", "YZ"}."YZ", "Display"=TRUE) -> (w349:T9)
              }
              frame "displayYZSum" {
                n131 = Unbundle By Name(w361) -> ("PythonSession"=w355:refnum<k35>)
                n132 = call "HoloPy_sum_YZ_planes_from_volume.vi"("error in (no error)"=w357, "Refnum in"=w355) -> ("error out"=w356:errorcluster, "YZ Plane"=w354:sgl[][])  [unwired: 7 in, 1 out]
                n133 = Bundle By Name(cluster=w361, "LabelPicture"="Volume YZ sum plane" ("Label.Text"), "Display"=w354, "planeToDisplayFeatures"=enum16{"XY", "XZ", "YZ"}."YZ", "Display"=TRUE) -> (w360:T9)
              }
              frame "displaySubVolume" {
                n134 = Unbundle By Name(w376) -> ("PythonSession"=w371:refnum<k35>)
                n135 = Variant To Data(error in=w369, type=T7 {"X"=0, "Y"=0, "Z"=0, "XYsize"=0, "ZSize"=0} ("param"), Variant=w368) -> (data=w366:T7, error out=w365:errorcluster)
                n136 = call "HoloPy_subvolume_3planes.vi"("error in (no error)"=w365, "param"=w366, "Refnum in"=w371) -> ("error out"=w372:errorcluster, "YZ Plane"=w370:sgl[][])  [unwired: 6 in, 1 out]
                n137 = Bundle By Name(cluster=w376, "LabelPicture"="sub volume 3 planes" ("Label.Text"), "Display"=w370, "planeToDisplayFeatures"=enum16{"XY", "XZ", "YZ"}."XY", "Display"=TRUE) -> (w375:T9)
              }
              frame "displayHolo_plane" {
                w383 = u16 0 ("Plane number")
                (unwired) "Hologram plane" ("Label.Text")
                n138 = Variant To Data(error in=w394, type=w383, Variant=w393) -> (data=w390:u16, error out=w392:errorcluster)
                n139 = Unbundle By Name(w389) -> ("PythonSession"=w391:refnum<k35>)
                n140 = call "HoloPy_get_reconstruction_plane.vi"("error in (no error)"=w392, "plane number"=w390, "Refnum in"=w391) -> ("error out"=w381:errorcluster, "HOLO_array"=w386:sgl[][])  [unwired: 6 in, 1 out]
                n141 = Number To Decimal String(number=w383) -> (decimal integer string=w382:string)  [unwired: 1 in]
                n142 = Concatenate Strings("Hologram plane number " ("Label.Text"), w382) -> (w384:string)
                n143 = Bundle By Name(cluster=w389, "LabelPicture"=w384, "Display"=w386, "planeToDisplayFeatures"=enum16{"XY", "XZ", "YZ"}."XY", "Display"=TRUE) -> (w388:T9)
              }
              frame "displayBin_plane" {
                w404 = u16 0 ("Plane number")
                n144 = Variant To Data(error in=w411, type=w404, Variant=w410) -> (data=w401:u16, error out=w402:errorcluster)
                n145 = Unbundle By Name(w409) -> ("PythonSession"=w400:refnum<k35>)
                n146 = call "HoloPy_get_binarised_plane.vi"("error in (no error)"=w402, "plane number"=w401, "Refnum in"=w400) -> ("error out"=w398:errorcluster, "HOLO_array"=w399:sgl[][])  [unwired: 6 in, 1 out]
                n147 = Number To Decimal String(number=w404) -> (decimal integer string=w403:string)  [unwired: 1 in]
                n148 = Concatenate Strings("Hologram bin plane number " ("Label.Text"), w403) -> (w405:string)
                n149 = Bundle By Name(cluster=w409, "LabelPicture"=w405, "Display"=w399, "planeToDisplayFeatures"=enum16{"XY", "XZ", "YZ"}."XY", "Display"=TRUE) -> (w408:T9)
              }
              frame "TEST SUM BIN PLANE" {
                n150 = Unbundle By Name(w422) -> ("PythonSession"=w416:refnum<k35>)
                n151 = call "HoloPy_get_sum_bin_planes.vi"("error in (no error)"=w415, "Refnum in"=w416) -> ("error out"=w419:errorcluster, "XY Plane"=w418:i32[][])  [unwired: 7 in, 1 out]
                n152 = To Single Precision Float(number=w418) -> (single precision float=w417:sgl[][])
                n153 = Bundle By Name(cluster=w422, "LabelPicture"="Sum thresholded planes" ("Label.Text"), "Display"=w417, "Display"=TRUE) -> (w421:T9)
              }
              frame "start batch" {
                n154 = Variant To Data(error in=w433, type=T6 {"Display real-time results"=FALSE, "Remove mean Hologram"=FALSE, "Binarisation thresold "=enum."compute on 1st hologram"} ("Batch parameters"), Variant=w432) -> (data=w428:T6, error out=w431:errorcluster)
                n155 = call "batchQueuesCommands.vi"(7:w425, "error in (no error)"=w431, "Batch parameters"=w428, 10:w427, "QueueMessages"=w434) -> ("error out"=w429:errorcluster)  [unwired: 6 in]
                n156 = Bundle By Name(cluster=w425, "BATCH?"=TRUE ("reconstructed?")) -> (w424:T9)
              }
              frame "cancelBatch" {
                w436 = FALSE ("BATCH?")
                w440 = sgl[][] [] ("Holo")
                n157 = Unbundle By Name(w451) -> ("PythonOpen?"=w450:bool, "PythonSession"=w449:refnum<k35>)
                n158 = Flush Queue(queue=w444, error in (no error)=w443) -> (error out=w442:errorcluster)  [unwired: 2 out]
                n159 = case shown="True" w450 {
                  tunnel: w442 -> [w454 w457]
                  tunnel: w449 -> [_ w456]
                  tunnel: [w454 w455] -> w438
                  frame False {
                  }
                  frame True {
                    n160 = Close Python Session(session in=w456, error in=w457) -> (11:w455:errorcluster)
                  }
                }
                n161 = Bundle By Name(cluster=w451, "TEST?"=w436, "BATCH?"=w436, "Status"="batch canceled" ("command"), "PythonSession"=refnum<k35> refnum, "PythonOpen?"=FALSE ("allocated?"), "Display"=w440, "FEATURES(µm)"=w440, "Holo parameters"=T5 {"wavelength"=0.0, "optical index"=0.0, "Holo size X"=0, "Holo size Y"=0, "pixel size"=0.0, "objective magnification"=0.0}, "Analyse parameters"=T3 {"propagation"={"distance ini"=0.0, "number of planes"=0, "step"=0.0, "Fourier BP filter (pix)"={"High pass (0=none)"=0.0, "Low Pass (0=none)"=0.0}}, "Focus"={"Type"=enum."SUM_OF_INTENSITY", "Sum size"=1}, "Remove mean Hologram"=FALSE, "CCL parameters"={"Threshold ( N x Standard deviation)"=10.0, "Connectivity"=enum."26", "min voxel"=1.0, "max voxel"=0.0}}, "LIST HOLO BATCH"=path[] []) -> (w452:T9)
              }
              frame "savePosition" {
                n162 = Variant To Data(error in=w467, type=path "" ("Holograms directory"), Variant=w466) -> (data=w461:path, error out=w464:errorcluster)
                n163 = Unbundle By Name(w460) -> ("PythonSession"=w462:refnum<k35>, "FEATURES(µm)"=w459:sgl[][])
                n164 = call "HoloPy_save_Features_csv.vi"("error in (no error)"=w464, "path csv file"=w461, "Array"=w459, "Refnum in"=w462) -> ("error out"=w463:errorcluster)  [unwired: 6 in, 1 out]
              }
              frame "EXIT" {
                w469 = FALSE ("allocated?")
                n165 = Unbundle By Name(w471) -> ("PythonOpen?"=w477:bool, "PythonSession"=w475:refnum<k35>)
                n166 = case shown="True" w477 {
                  tunnel: w476 -> [w481 w484]
                  tunnel: w475 -> [_ w483]
                  tunnel: [w481 w482] -> w474
                  frame False {
                  }
                  frame True {
                    n167 = Close Python Session(session in=w483, error in=w484) -> (11:w482:errorcluster)
                  }
                }
                n168 = Generate User Event(user event=w479, event data cluster=TRUE ("event data"), error in=w474) -> (error out=w473:errorcluster)  [unwired: 1 in, 1 out]
                n169 = Bundle By Name(cluster=w471, "PythonOpen?"=w469, "TEST?"=w469, "BATCH?"=w469) -> (w470:T9)
              }
            }
            n170 = call "displayMessageSender.vi"("error in (no error)"=w76, "DatasIN"=w79, "QueueMsgIN"=w78) -> ("error out"=w77:errorcluster, "DatasOUT"=w75:T9)  [unwired: 6 in, 1 out]
          }
          frame Error {
            n171 = flat-sequence {
              tunnel: w490 -> [w492]
              tunnel: w489 -> [w493]
              tunnel: [w493] -> w488
              tunnel: w488 -> [w495]
              frame #0 {
                n172 = Flush Queue(queue=w492) -> (queue out=w491:refnum<queue>)  [unwired: 1 in, 2 out]
                n173 = Enqueue Element(queue=w491, element=cluster{"command":string, "data":variant} {"command"="freeGPU", "data"=variant}) -> ()  [unwired: 2 in, 3 out]
              }
              frame #1 {
                n174 = call <vilib>:"Simple Error Handler.vi"("error in (no error)"=w495) -> ()  [unwired: 4 in, 5 out]
              }
            }
          }
        }
      }
      n175 = while {
        tunnel: w66 -> [w499]
        tunnel: w65 -> [w498]
        tunnel: [w497] -> w64
        tunnel: w61 -> [w496]
        stop <- w500 stop-if-true
        # "USER EVENT"
        n176 = event shown="[3] \"openHOLO\": Value Change" {
          selector: w498 -> [_ _ _ _ _ _ _ _ _ _ _ _ _ _ _ _ _ _ _ _ _ _]
          dyn-events: _ -> [_ _ _ _ _ _ _ _ _ _ _ _ _ _ _ _ _ _ _ _ _ _]
          timeout: _ -> [_ _ _ _ _ _ _ _ _ _ _ _ _ _ _ _ _ _ _ _ _ _]
          tunnel: [FALSE FALSE TRUE _ _ _ _ _ _ _ _ _ _ _ _ _ _ _ _ _ _ _] -> w500
          tunnel: w499 -> [w505 w513 _ w533 w546 w548 w554 w557 w560 w563 w566 w569 w572 w577 w582 w587 w590 w593 w599 w603 w608 w624]
          tunnel: [w501 w512 _ w534 w541 w550 w555 w558 w561 w564 w567 w570 w573 w578 w583 w588 w591 w594 w602 _ _ _] -> w497
          tunnel: w496 -> [w503 w507 _ _ _ w547 _ _ _ _ _ _ _ _ _ _ _ _ _ _ _ _]
          event "EXIT": Value Change {
            w504 = cluster{"command":string, "data":variant} {"command"="EXIT", "data"=variant} ("element")
            n177 = event-data() -> ()  [unwired: 1 in, 1 out]
            n178 = Enqueue Element(queue=w505, element=w504) -> (error out=w502:errorcluster)  [unwired: 2 in, 2 out]
            n179 = Enqueue Element(queue=w503, element=w504, error in (no error)=w502) -> (error out=w501:errorcluster)  [unwired: 1 in, 2 out]
          }
          event Panel Close? {
            n180 = event-data() -> ()  [unwired: 1 in, 4 out]
            n181 = Two Button Dialog(message="EXIT APPLICATION?", 2:"YES" ("T button name (\"OK\")")) -> (T button?=w509:bool)  [unwired: 1 in]
            n182 = case shown="True" w509 {
              tunnel: w513 -> [_ w520]
              tunnel: [errorcluster {"status"=FALSE, "code"=0, "source"=""} ("error out") w516] -> w512
              tunnel: w507 -> [_ w518]
              frame False {
              }
              frame True {
                w517 = cluster{"command":string, "data":variant} {"command"="EXIT", "data"=variant} ("element")
                n183 = Enqueue Element(queue=w520, element=w517) -> (error out=w519:errorcluster)  [unwired: 2 in, 2 out]
                n184 = Enqueue Element(queue=w518, element=w517, error in (no error)=w519) -> (error out=w516:errorcluster)  [unwired: 1 in, 2 out]
              }
            }
            n185 = event-data("Discard?"=TRUE) -> ()  [unwired: 1 in, 1 out]
          }
          event User Event {
            n186 = event-data() -> ()  [unwired: 1 in, 5 out]
          }
          event "openHOLO": Value Change {
            (unwired) T11 {"Test hologram path"=path "", "Display?"=FALSE} ("openHolo")
            w528 = TRUE  # Display?
            n187 = event-data() -> ()  [unwired: 1 in, 1 out]
            n188 = local read "Holo parameters"() -> (w522:T5)
            n189 = local read "Analyse parameters"() -> (w523:T3)
            n190 = local read item#-1() -> (w525)
            n191 = Bundle(cluster=T10 {"Holo parameters"={"wavelength"=0.0, "optical index"=0.0, "Holo size X"=0, "Holo size Y"=0, "pixel size"=0.0, "objective magnification"=0.0}, "Analyse parameters"={"propagation"={"distance ini"=0.0, "number of planes"=0, "step"=0.0, "Fourier BP filter (pix)"={"High pass (0=none)"=0.0, "Low Pass (0=none)"=0.0}}, "Focus"={"Type"=enum."SUM_OF_INTENSITY", "Sum size"=0}, "Remove mean Hologram"=FALSE, "CCL parameters"={"Threshold ( N x Standard deviation)"=10.0, "Connectivity"=enum."26", "min voxel"=1.0, "max voxel"=0.0}}} ("Parameters"), w522, w523, w525) -> (w529:T10)
            n192 = Bundle By Name(cluster=cluster{"command":string, "data":variant} {"command"="allocate", "data"=variant} ("element"), "data"=w529) -> (w530:cluster{"command":string, "data":variant})
            n193 = Bundle("Test hologram path"="Test hologram path", "Display?"=w528) -> (w526:T11)  [unwired: 1 in]
            n194 = Enqueue Element(queue=w533, element=w530) -> (queue out=w532:refnum<queue>)  [unwired: 2 in, 2 out]
            n195 = Bundle By Name(cluster=cluster{"command":string, "data":variant} {"command"="openHolo", "data"=variant} ("element"), "data"=w526) -> (w535:cluster{"command":string, "data":variant})
            n196 = Enqueue Element(queue=w532, element=w535) -> (error out=w534:errorcluster)  [unwired: 2 in, 2 out]
          }
          event "removeMeanHolo": Value Change {
            w538 = TRUE  # display?
            n197 = event-data() -> ()  [unwired: 1 in, 1 out]
            n198 = Bundle By Name(cluster=cluster{"command":string, "data":variant} {"command"="computeMeanHolo", "data"=variant} ("element"), "data"="Holograms directory") -> (w544:cluster{"command":string, "data":variant})
            n199 = Enqueue Element(queue=w546, element=w544) -> (queue out=w542:refnum<queue>, error out=w543:errorcluster)  [unwired: 2 in, 1 out]
            n200 = Bundle By Name(cluster=cluster{"command":string, "data":variant} {"command"="removeMeanHolo", "data"=variant} ("element"), "data"=w538) -> (w539:cluster{"command":string, "data":variant})
            n201 = Enqueue Element(queue=w542, element=w539, error in (no error)=w543) -> (error out=w541:errorcluster)  [unwired: 1 in, 2 out]
          }
          event "close HOLO": Value Change {
            n202 = event-data() -> ()  [unwired: 1 in, 1 out]
            n203 = Enqueue Element(queue=w547, element=cluster{"command":string, "data":variant} {"command"="closeHolo", "data"=variant}) -> (error out=w551:errorcluster)  [unwired: 2 in, 2 out]
            n204 = Enqueue Element(queue=w548, element=cluster{"command":string, "data":variant} {"command"="freeGPU", "data"=variant}, error in (no error)=w551) -> (error out=w550:errorcluster)  [unwired: 1 in, 2 out]
          }
          event "reconstruct&Focus": Value Change {
            n205 = event-data() -> ()  [unwired: 1 in, 1 out]
            n206 = Enqueue Element(queue=w554, element=cluster{"command":string, "data":variant} {"command"="reconstructAndFocus", "data"=variant}) -> (error out=w555:errorcluster)  [unwired: 2 in, 2 out]
          }
          event "displayXYMax": Value Change {
            n207 = event-data() -> ()  [unwired: 1 in, 1 out]
            n208 = Enqueue Element(queue=w557, element=cluster{"command":string, "data":variant} {"command"="displayXYMax", "data"=variant}) -> (error out=w558:errorcluster)  [unwired: 2 in, 2 out]
          }
          event "display_XY_SUM": Value Change {
            n209 = event-data() -> ()  [unwired: 1 in, 1 out]
            n210 = Enqueue Element(queue=w560, element=cluster{"command":string, "data":variant} {"command"="displayXYSum", "data"=variant}) -> (error out=w561:errorcluster)  [unwired: 2 in, 2 out]
          }
          event "display_XZ_SUM": Value Change {
            n211 = event-data() -> ()  [unwired: 1 in, 1 out]
            n212 = Enqueue Element(queue=w563, element=cluster{"command":string, "data":variant} {"command"="displayXZSum", "data"=variant}) -> (error out=w564:errorcluster)  [unwired: 2 in, 2 out]
          }
          event "display_YZ_SUM": Value Change {
            n213 = event-data() -> ()  [unwired: 1 in, 1 out]
            n214 = Enqueue Element(queue=w566, element=cluster{"command":string, "data":variant} {"command"="displayYZSum", "data"=variant}) -> (error out=w567:errorcluster)  [unwired: 2 in, 2 out]
          }
          event "displayHolo": Value Change {
            n215 = event-data() -> ()  [unwired: 1 in, 1 out]
            n216 = Enqueue Element(queue=w569, element=cluster{"command":string, "data":variant} {"command"="displayHolo", "data"=variant}) -> (error out=w570:errorcluster)  [unwired: 2 in, 2 out]
          }
          event "TEST SUM BIN PLANE": Value Change {
            n217 = event-data() -> ()  [unwired: 1 in, 1 out]
            n218 = Enqueue Element(queue=w572, element=cluster{"command":string, "data":variant} {"command"="TEST SUM BIN PLANE", "data"=variant}) -> (error out=w573:errorcluster)  [unwired: 2 in, 2 out]
          }
          event "displayPlane": Value Change {
            n219 = event-data() -> ()  [unwired: 1 in, 6 out]
            n220 = Bundle By Name(cluster=cluster{"command":string, "data":variant} {"command"="displayHolo_plane", "data"=variant} ("element"), "data"="Plane number") -> (w575:cluster{"command":string, "data":variant})
            n221 = Enqueue Element(queue=w577, element=w575) -> (error out=w578:errorcluster)  [unwired: 2 in, 2 out]
          }
          event "display\nsub-volume\n3 planes": Value Change {
            n222 = event-data() -> ()  [unwired: 1 in, 6 out]
            n223 = Bundle By Name(cluster=cluster{"command":string, "data":variant} {"command"="displaySubVolume", "data"=variant} ("element"), "data"="param") -> (w580:cluster{"command":string, "data":variant})
            n224 = Enqueue Element(queue=w582, element=w580) -> (error out=w583:errorcluster)  [unwired: 2 in, 2 out]
          }
          event "displayBinPlane": Value Change {
            n225 = event-data() -> ()  [unwired: 1 in, 6 out]
            n226 = local read "Plane number"() -> (w584:u16)
            n227 = Bundle By Name(cluster=cluster{"command":string, "data":variant} {"command"="displayBin_plane", "data"=variant} ("element"), "data"=w584) -> (w585:cluster{"command":string, "data":variant})
            n228 = Enqueue Element(queue=w587, element=w585) -> (error out=w588:errorcluster)  [unwired: 2 in, 2 out]
          }
          event "displayXZMax": Value Change {
            n229 = event-data() -> ()  [unwired: 1 in, 1 out]
            n230 = Enqueue Element(queue=w590, element=cluster{"command":string, "data":variant} {"command"="displayXZMax", "data"=variant}) -> (error out=w591:errorcluster)  [unwired: 2 in, 2 out]
          }
          event "displayYZMax": Value Change {
            n231 = event-data() -> ()  [unwired: 1 in, 1 out]
            n232 = Enqueue Element(queue=w593, element=cluster{"command":string, "data":variant} {"command"="displayYZMax", "data"=variant}) -> (error out=w594:errorcluster)  [unwired: 2 in, 2 out]
          }
          event "findFeatures": Value Change {
            n233 = event-data() -> ()  [unwired: 1 in, 1 out]
            n234 = Enqueue Element(queue=w599, element=cluster{"command":string, "data":variant} {"command"="computeThreshold", "data"=variant}) -> (queue out=w598:refnum<queue>, error out=w597:errorcluster)  [unwired: 2 in, 1 out]
            n235 = Bundle By Name(cluster=cluster{"command":string, "data":variant} {"command"="findFeatures", "data"=variant} ("element"), "data"=cluster{"imageNumber":u32, "Display":bool} {"imageNumber"=0, "Display"=TRUE}) -> (w600:cluster{"command":string, "data":variant})
            n236 = Enqueue Element(queue=w598, element=w600, error in (no error)=w597) -> (error out=w602:errorcluster)  [unwired: 1 in, 2 out]
          }
          event #19 (no event record) {
            n237 = event-data() -> ()  [unwired: 1 in, 6 out]
            n238 = Bundle By Name(cluster=cluster{"command":string, "data":variant} {"command"="updateCCLparam", "data"=variant} ("element")) -> (w605:cluster{"command":string, "data":variant}, "data"=w604:variant)
            n239 = Enqueue Element(queue=w603, element=w605) -> ()  [unwired: 2 in, 3 out]
          }
          event "BATCH": Value Change {
            n240 = event-data() -> ()  [unwired: 1 in, 1 out]
            n241 = local read "Holograms directory"() -> (w615:path)
            n242 = Bundle(cluster=T10 {"Holo parameters"={"wavelength"=0.0, "optical index"=0.0, "Holo size X"=0, "Holo size Y"=0, "pixel size"=0.0, "objective magnification"=0.0}, "Analyse parameters"={"propagation"={"distance ini"=0.0, "number of planes"=0, "step"=0.0, "Fourier BP filter (pix)"={"High pass (0=none)"=0.0, "Low Pass (0=none)"=0.0}}, "Focus"={"Type"=enum."SUM_OF_INTENSITY", "Sum size"=0}, "Remove mean Hologram"=FALSE, "CCL parameters"={"Threshold ( N x Standard deviation)"=10.0, "Connectivity"=enum."26", "min voxel"=1.0, "max voxel"=0.0}}} ("Parameters"), "Holo parameters"="Holo parameters", "Analyse parameters"="Analyse parameters") -> (w620:T10)
            n243 = Enqueue Element(queue=w608) -> (queue out=w607:refnum<queue>)  [unwired: 3 in, 2 out]
            n244 = Bundle By Name(cluster=cluster{"command":string, "data":variant} {"command"="allocate", "data"=variant} ("element"), "data"=w620) -> (w622:cluster{"command":string, "data":variant})
            n245 = Enqueue Element(queue=w607, element=w622) -> (queue out=w619:refnum<queue>)  [unwired: 2 in, 2 out]
            n246 = Bundle By Name(cluster=cluster{"command":string, "data":variant} {"command"="get holo path list", "data"=variant} ("element"), "data"=w615) -> (w616:cluster{"command":string, "data":variant})
            n247 = Enqueue Element(queue=w619, element=w616) -> (queue out=w618:refnum<queue>)  [unwired: 2 in, 2 out]
            n248 = Bundle By Name(cluster=cluster{"command":string, "data":variant} {"command"="start batch", "data"=variant} ("element"), "data"="Batch parameters") -> (w613:cluster{"command":string, "data":variant})
            n249 = Enqueue Element(queue=w618, element=w613) -> ()  [unwired: 2 in, 3 out]
          }
          event "CANCEL_BATCH": Value Change {
            n250 = event-data() -> ()  [unwired: 1 in, 6 out]
            n251 = Enqueue Element At Opposite End(queue=w624, element=cluster{"command":string, "data":variant} {"command"="cancelBatch", "data"=variant}) -> ()  [unwired: 2 in, 3 out]
          }
        }
      }
      n252 = while {
        tunnel: w61 -> [w633]
        tunnel: w63 -> [w627]
        tunnel: [w626] -> w60
        tunnel: w58 -> [w625]
        stop <- w628 stop-if-true
        # "DISPLAY AND SAVE"
        n253 = Dequeue Element(queue=w633) -> (element=w631:cluster{"command":string, "data":variant}, error out=w632:errorcluster)  [unwired: 2 in, 2 out]
        n254 = Unbundle(w631) -> ("command"=w630:string, "data"=w629:variant)
        n255 = case shown="\"updateLabelPicture\"" w630 {
          tunnel: w632 -> [w634 w641 w649 w667 w685 w686]
          tunnel: w629 -> [_ w640 w648 w666 w684 _]
          tunnel: [FALSE FALSE FALSE FALSE FALSE TRUE] -> w628
          tunnel: w627 -> [_ _ _ _ _ w688]
          tunnel: [w634 w637 w645 w660 w682 w686] -> w626
          tunnel: w625 -> [_ _ w643 _ _ _]
          frame "", Default {
          }
          frame "updateStatus" {
            n256 = Variant To Data(error in=w641, type="" ("return value"), Variant=w640) -> (data=→"Status":string, error out=w637:errorcluster)
          }
          frame "updateBtnIHM" {
            n257 = Variant To Data(error in=w649, type=T12 {"allocated?"=FALSE, "reconstructed?"=FALSE, "BATCH?"=FALSE} ("output cluster"), Variant=w648) -> (data=w642:T12, error out=w644:errorcluster)
            n258 = disable-structure shown="Disabled" {
              disable-tunnel: [w653 _] -> w645
              disable-tunnel: w644 -> [w652 _]
              disable-tunnel: w643 -> [w651 _]
              disable-tunnel: w642 -> [w650 _]
              frame Disabled {
                n259 = call "activateBtnIHM.vi"("error in (no error)"=w652, "State"=w650, "References"=w651) -> ("error out"=w653:errorcluster)  [unwired: 8 in]
              }
              frame Enabled {
              }
            }
          }
          frame "updateDisplay" {
            n260 = Variant To Data(error in=w667, type=T13 {"Holo"=[], "XYFeatures(pix)"=[], "FEATURES(µm)"=[]} ("output cluster"), Variant=w666) -> (data=w664:T13, error out=w661:errorcluster)
            n261 = Unbundle(w664) -> ("Holo"=w659:sgl[][], "XYFeatures(pix)"=w658:sgl[][], "FEATURES(µm)"=w656:sgl[][])
            "FEATURES" <- w656
            n262 = Not Equal?(x=w656, y=sgl[][] []) -> (x != y?=w655:bool)
            n263 = control-ref of="2D Picture"() -> (w662:refnum<vi>)
            n264 = call "convert_float_array_to_U8_Picture.vi"("Pict Refnum"=w662, "error in (no error)"=w661, "FEATURES (PIX)"=w658, "HOLO"=w659) -> ("error out"=w660:errorcluster, "new picture"=→"2D Picture":picture)  [unwired: 6 in]
            n265 = case shown="False" w655 {
              tunnel: w656 -> [_ w668]
              frame False {
              }
              frame True {
                w672 = 1000000.0
                n266 = Index Array(array=w668, index (col) #1=1 ("disabled index (col)"), index (col) #2=2 ("index (col)"), index (col) #3=3 ("index (col)")) -> (element #1=w673:sgl[], element #2=w674:sgl[], element #3=w675:sgl[])  [unwired: 3 in]
                n267 = Multiply(x=w674, y=w672) -> (x*y=w678:dbl[])
                n268 = Multiply(x=w673, y=w672) -> (x*y=w677:dbl[])
                n269 = Multiply(x=w675, y=w672) -> (x*y=w676:dbl[])
                n270 = call-poly <vilib>:"Plot Helper.vi"("z vector"=w676, "y vector"=w677, "x vector"=w678) -> ("3D Plot lvclass Array out"=→"3D Scatter":refnum<class "3D Plot Datatype.lvclass">[])  [unwired: 3 in, 5 out]
              }
            }
          }
          frame "updateLabelPicture" {
            n271 = Variant To Data(error in=w685, type="label" ("Label.Text"), Variant=w684) -> (data=w680:string, error out=w682:errorcluster)
            n272 = property on="2D Picture" class="Pict"("Caption.Text"=w680) -> ()  [unwired: 2 in, 2 out]
          }
          frame "EXIT" {
            n273 = Generate User Event(user event=w688, event data cluster=TRUE ("event data")) -> ()  [unwired: 2 in, 2 out]
          }
        }
      }
    }
    frame #2 {
      (unwired) "Volume XY max plane" ("Label.Text")
      n274 = Merge Errors(w691, w692, w693) -> (w690:errorcluster)
      n275 = Destroy User Event(user event=w694, error in=w690) -> (error out=w696:errorcluster)
      n276 = Unregister For Events(event registration refnum=w695, error in=w696) -> ()  [unwired: 1 out]
    }
  }
